vi "Close.vi"(8 "error in (no error)":errorcluster, 11 "PEU in":refnum<class "PEU.lvclass">) -> (0 "error out":errorcluster, 3 "PEU out":refnum<class "PEU.lvclass">)   [LabVIEW 2020, in "PEU.lvlib" / "PEU.lvclass"]
uses:
  PEU.lvclass
  PEU.lvclass/PEU.ctl
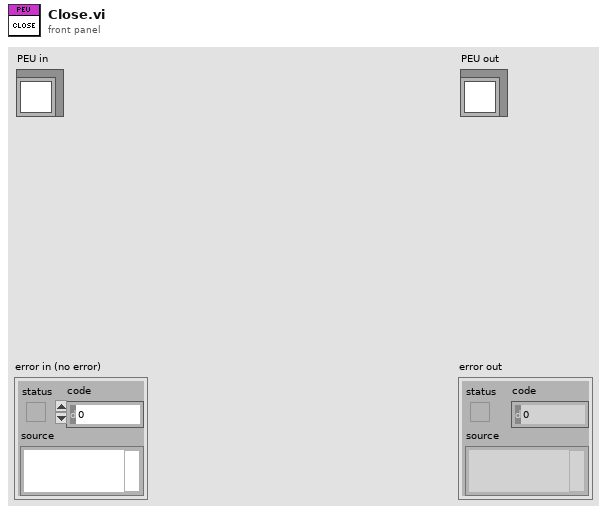
[diagram p1: front panel]
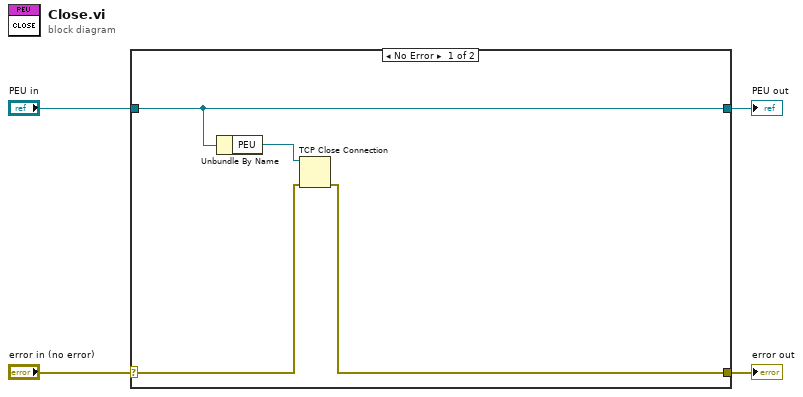
[diagram p0: block diagram]
diagram:
  n1 = case shown="No Error" "error in (no error)" {
    selector: "error in (no error)" -> [w6 w10]
    tunnel: [w5 w10] -> w3
    tunnel: [w8 w9] -> w1
    tunnel: "PEU in" -> [w8 w9]
    frame No Error {
      n2 = Unbundle By Name(w8) -> ("PEU"=w7:refnum<k5>)
      n3 = TCP Close Connection(connection ID=w7, error in (no error)=w6) -> (error out=w5:errorcluster)  [unwired: 1 in, 1 out]
    }
    frame Error {
    }
  }
  "error out" <- w3
  "PEU out" <- w1
